vi "Get Logging Timestamp in File Name.vi"(8 "error in":errorcluster, 11 "logging section":T1=18446744073709551615 format="%.0x") -> (0 "error out":errorcluster, 2 "timestamp in file name":bool, 3 "logging section out":T1 format="%.0x")   [LabVIEW 2020, in "AIM MIL-STD-1553 Scripting.lvlib"]
doc: "Returns whether the log file name will be modified to contain a timestamp."
uses:
  AIM MIL-STD-1553 Scripting.lvlib
  <vilib>/NI VeriStand/Custom Device API/Custom Device Item Ref.ctl
  Constants.vi
  <vilib>/NI VeriStand/Custom Device API/Get Item Property (Boolean).vi
  <vilib>/NI VeriStand/Custom Device API/Custom Device API.lvlib
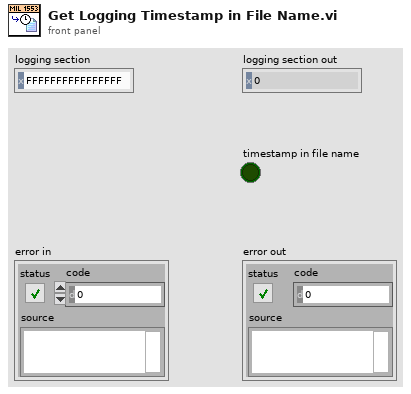
[diagram p1: front panel]
types:
  T1 = typedef "Custom Device API.lvlib/Custom Device Item Ref.ctl" = u64
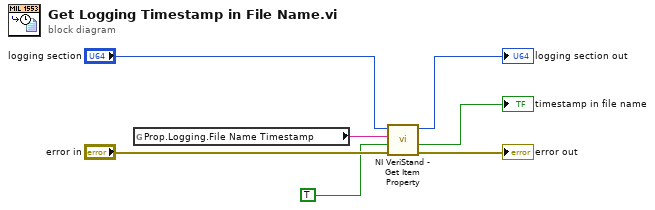
[diagram p0: block diagram]
diagram:
  n1 = global read "Constants.vi" "Prop.Logging.File Name Timestamp"() -> (w1:string)
  n2 = call-poly <vilib>:"NI VeriStand - Get Item Property.vi"("error in (no error)"="error in", "Default Value"=TRUE, "Property Name"=w1, "Item Ref in"="logging section") -> ("error out"=→"error out":errorcluster, "Value"=→"timestamp in file name":bool, "Item Ref out"=→"logging section out":T1)  [unwired: 4 in, 1 out]
